vi "Excel_New_Page.vi"(0 "Excel._Worksheet":refnum<k7>, 7 "name (Excel)":string, 9 "position (Excel)":cluster{"row":i32, "column":i32}, 11 "error in (no error)":errorcluster) -> (15 "error out":errorcluster)   [LabVIEW 2017, in "NI_ReportGenerationToolkit.lvlib"]
uses:
  <vilib>/addons/_office/NI_ReportGenerationToolkit.lvlib
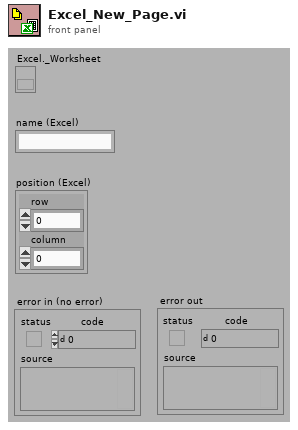
[diagram p1: front panel]
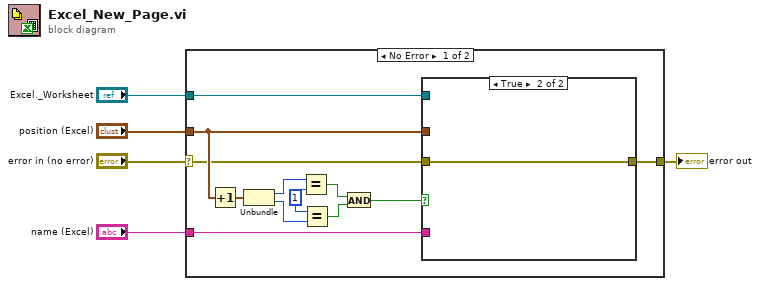
[diagram p0: block diagram]
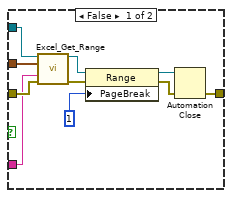
[diagram p2: hidden frame]
diagram:
  n1 = case shown="No Error" "error in (no error)" {
    selector: "error in (no error)" -> [w6 w29]
    tunnel: [w16 w29] -> w5
    tunnel: "Excel._Worksheet" -> [w9 _]
    tunnel: "name (Excel)" -> [w8 _]
    tunnel: "position (Excel)" -> [w7 _]
    frame No Error {
      w12 = 1
      n2 = Increment(x=w7) -> (x+1=w17:cluster{"row":i32, "column":i32})
      n3 = Unbundle(w17) -> ("row"=w14:i32, "column"=w13:i32)
      n4 = Equal?(x=w14, y=w12) -> (x = y?=w10:bool)
      n5 = Equal?(x=w12, y=w13) -> (x = y?=w11:bool)
      n6 = And(x=w10, y=w11) -> (x .and. y?=w15:bool)
      n7 = case shown="True" w15 {
        tunnel: [w26 w28] -> w16
        tunnel: w6 -> [w21 w28]
        tunnel: w9 -> [w20 _]
        tunnel: w8 -> [w18 _]
        tunnel: w7 -> [w19 _]
        frame False {
          n8 = call <vilib>:"Excel_Get_Range.vi"("Excel._Worksheet"=w20, "start"=w19, "name"=w18, "error in (no error)"=w21) -> ("Range"=w22:refnum<k7>, "error out"=w23:errorcluster)  [unwired: 1 in, 9 out]
          n9 = property class="Range"(reference=w22, error in=w23, "PageBreak"=1) -> (reference out=w25:refnum<k7>, error out=w24:errorcluster)
          n10 = Automation Close(3:w24, 5:w25) -> (0:w26:errorcluster)
        }
        frame True {
        }
      }
    }
    frame Error {
    }
  }
  "error out" <- w5
